vi "Log Change Connection.vi"(8 "error in (no error)":errorcluster, 11 "Server in":refnum<class "Server.lvclass">) -> (0 "error out":errorcluster, 3 "Server out":refnum<class "Server.lvclass">)   [LabVIEW 2018, in "Server.lvclass"]
uses:
  Server.lvclass
  Server.lvclass/Server.ctl
  Comm/Stream/Stream.lvclass
  Log/Log.lvclass
panel:
  out "current time":timestamp
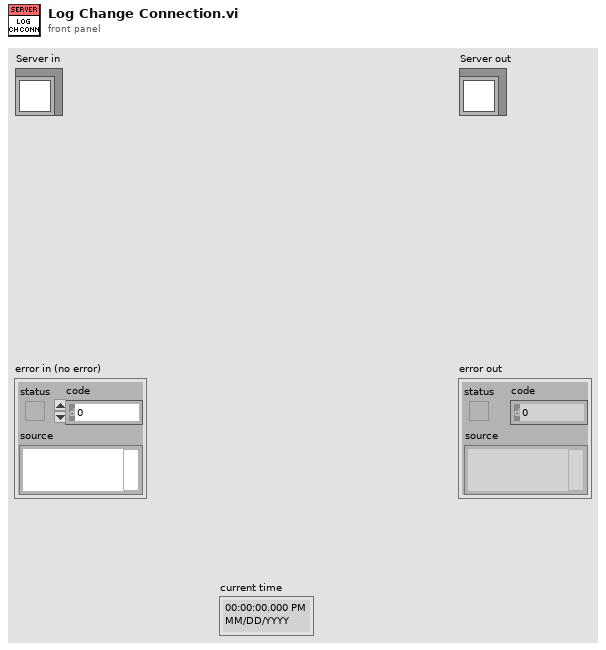
[diagram p1: front panel]
types:
  T1 = enum16{"INFO ", "TRACE", "DEBUG", "WARN ", "ERROR", "FATAL", "OTHER"}
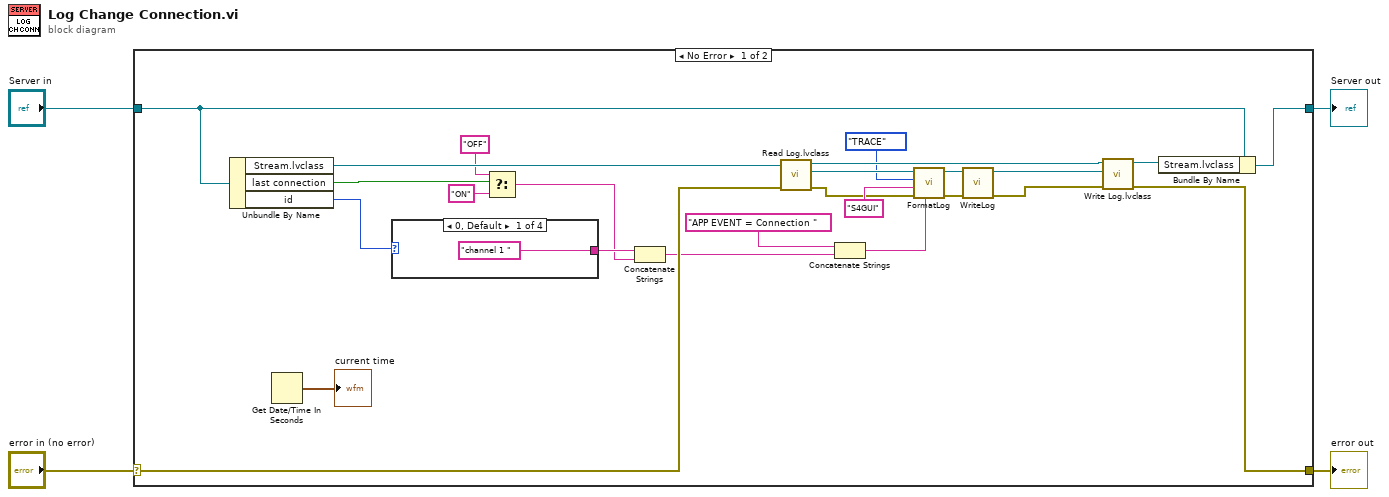
[diagram p0: block diagram]
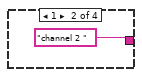
[diagram p2: hidden frame]
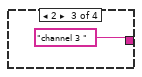
[diagram p3: hidden frame]
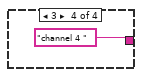
[diagram p4: hidden frame]
diagram:
  n1 = case shown="No Error" "error in (no error)" {
    selector: "error in (no error)" -> [w17 w35]
    tunnel: [w18 w35] -> w3
    tunnel: [w25 w34] -> w1
    tunnel: "Server in" -> [w29 w34]
    frame No Error {
      n2 = Unbundle By Name(w29) -> ("Stream.lvclass"=w28:refnum<class "Stream.lvclass">, "last connection"=w23:bool, "id"=w24:u32)
      n3 = Get Date/Time In Seconds() -> (seconds since 1Jan1904=→"current time":timestamp)
      n4 = case shown="0, Default" w24 {
        tunnel: ["channel 1 " ("string") "channel 2 " ("string") "channel 3 " ("string") "channel 4 " ("string")] -> w20
        frame 0, Default {
        }
        frame 1 {
        }
        frame 2 {
        }
        frame 3 {
        }
      }
      n5 = Select(t="OFF" ("string"), s=w23, f="ON" ("string")) -> (s? t:f=w19:string)
      n6 = Concatenate Strings(w20, w19) -> (w9:string)
      n7 = call-dynamic "Read Log.lvclass.vi"("error in (no error)"=w17, "Comm in"=w28) -> ("error out"=w7:errorcluster, "Log.lvclass"=w12:refnum<class "Log.lvclass">, "Comm out"=w27:refnum<class "Stream.lvclass">)  [unwired: 7 in]
      n8 = Concatenate Strings("APP EVENT = Connection " ("string"), w9) -> (w8:string)
      n9 = call-dynamic "FormatLog.vi"("log input"=w8, "error in (no error)"=w7, "System"="S4GUI", "Type"=T1."TRACE", "Log in"=w12) -> ("error out"=w14:errorcluster, "Log out"=w15:refnum<class "Log.lvclass">)  [unwired: 5 in]
      n10 = call-dynamic "WriteLog.vi"("error in (no error)"=w14, "Log in"=w15) -> ("error out"=w10:errorcluster, "Log out"=w11:refnum<class "Log.lvclass">)  [unwired: 8 in]
      n11 = call-dynamic "Write Log.lvclass.vi"("error in (no error)"=w10, "Log.lvclass"=w11, "Comm in"=w27) -> ("error out"=w18:errorcluster, "Comm out"=w26:refnum<class "Stream.lvclass">)  [unwired: 7 in]
      n12 = Bundle By Name(cluster=w29, "Stream.lvclass"=w26) -> (w25:refnum<class "Server.lvclass">)
    }
    frame Error {
    }
  }
  "error out" <- w3
  "Server out" <- w1
